vi "image_avg.vi"(10 "points / pixel":i32, 11 "input array":dbl[][](array[numeric])) -> (3 "output array":dbl[][](array[numeric]))   [LabVIEW 2013]
panel:
  out "after intial reshape":dbl[][](array[numeric])
  out "before final reshape":dbl[][](array[numeric])
  out "dim 2":i32
  out "dim 1":i32
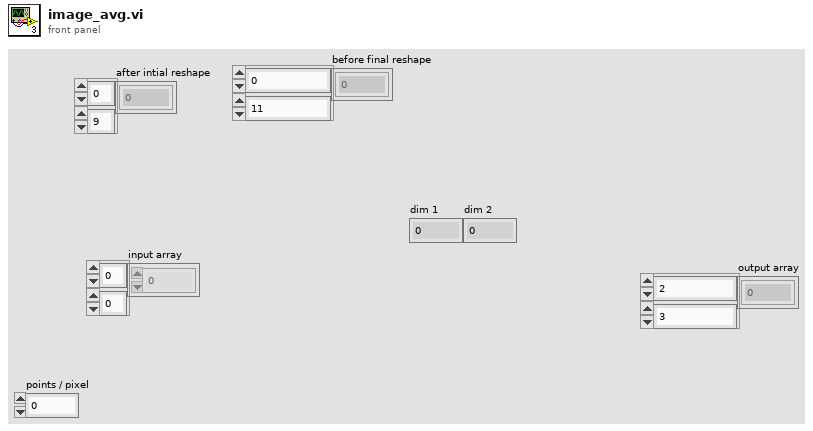
[diagram p1: front panel]
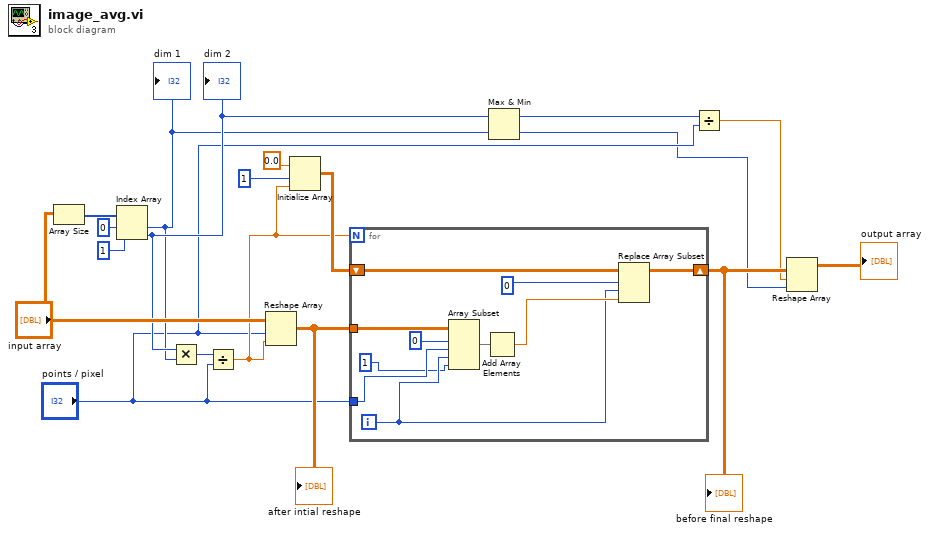
[diagram p0: block diagram]
diagram:
  n1 = Array Size(array="input array") -> (size(s)=w13:i32[])
  n2 = Index Array(array=w13, index #1=0 ("index"), index #2=1 ("index")) -> (element #1=w5:i32, element #2=w6:i32)
  "dim 1" <- w5
  "dim 2" <- w6
  n3 = Multiply(x=w6, y=w5) -> (x*y=w10:i32)
  n4 = Divide(x=w10, y="points / pixel") -> (x/y=w9:dbl)
  n5 = Reshape Array("input array", "points / pixel", w9) -> (w18:dbl[][])
  "after intial reshape" <- w18
  n6 = Initialize Array(0.0 ("element"), 1 ("dimension size"), w9) -> (w15:dbl[][])
  n7 = for {
    N: w9 -> [_]
    tunnel: w18 -> [w28]
    shift-right: [w25] -> w8
    shift-left: w15 -> [w24]
    tunnel: "points / pixel" -> [w20]
    i -> [w21]
    n8 = Array Subset(array=w28, index (row)=0 ("index"), length (row)=w20, index (col)=w21, length (col)=1 ("length")) -> (w26:dbl[][])
    n9 = Add Array Elements(numeric array=w26) -> (sum=w22:dbl)
    n10 = Replace Array Subset(array=w24, new element=w22, index (row)=0 ("length"), index (col)=w21) -> (w25:dbl[][])
  }
  "before final reshape" <- w8
  n11 = Max & Min(x=w6, y=w5) -> (max(x,y)=w4:i32, min(x,y)=w1:i32)
  n12 = Divide(x=w4, y="points / pixel") -> (x/y=w2:dbl)
  n13 = Reshape Array(w8, w2, w1) -> (→"output array":dbl[][])
